vi "API - Stream - Start Data Streaming from Device.vi"(8 "error in":errorcluster, 10 "Streaming Rate (Hz)":i32, 11 "DAQiFi Device Properties In":T1) -> (0 "error out":errorcluster, 3 "DAQiFi Device Properties Out":T1)   [LabVIEW 2021]
doc: "Send a command to start the streaming of data from the DAQ device."
uses:
  TypeDefs/TypeDef - Cluster of DAQiFi Device Properties.ctl
  TypeDefs/Enum - Connection Type.ctl
  TCP - Asynchronous Write.vi
  USB - Asynchronous Write.vi
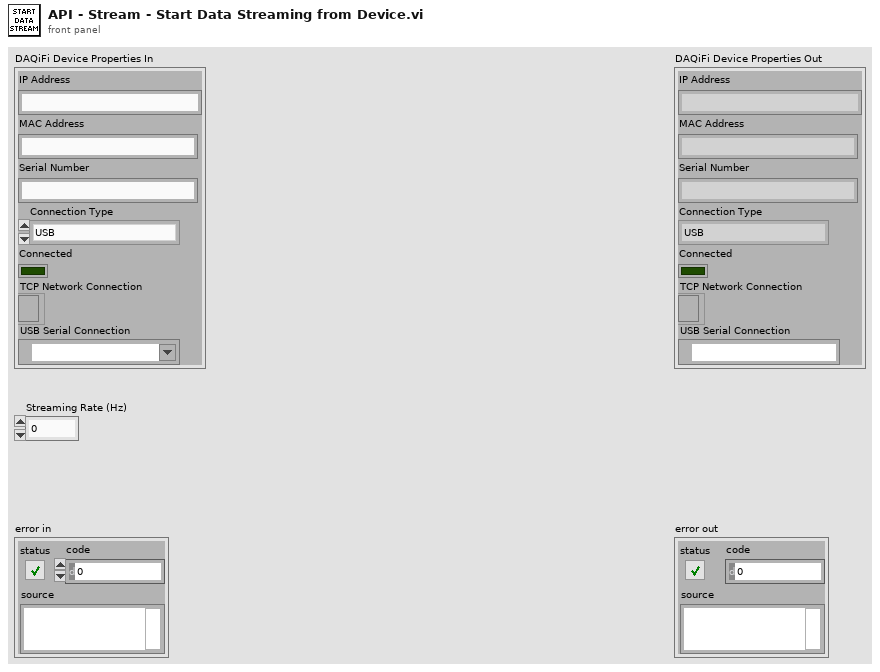
[diagram p1: front panel]
types:
  T1 = typedef "TypeDef - Cluster of DAQiFi Device Properties.ctl" = cluster{"IP Address":string, "MAC Address":string, "Serial Number":string, "Connection Type":T2, "Connected":bool, "TCP Network Connection":refnum<k5>, "USB Serial Connection":refnum<visa-resource-name>}
  T2 = typedef "Enum - Connection Type.ctl" = enum16{"USB", "TCP"}
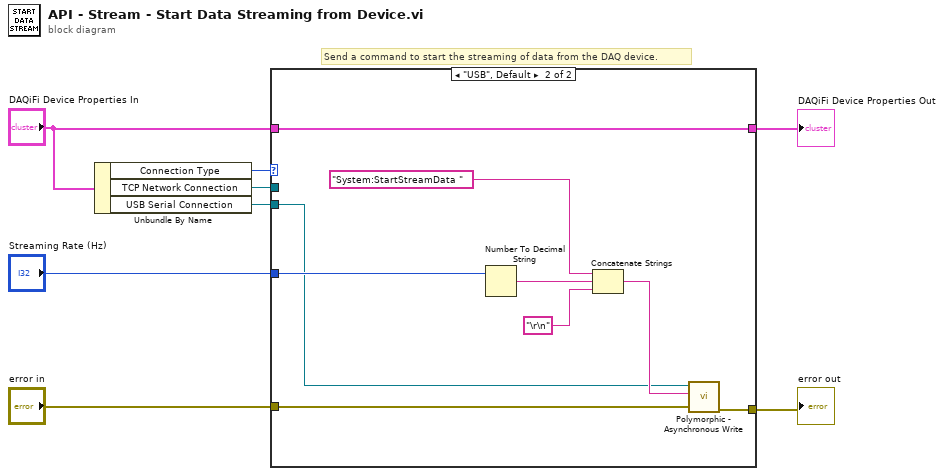
[diagram p0: block diagram]
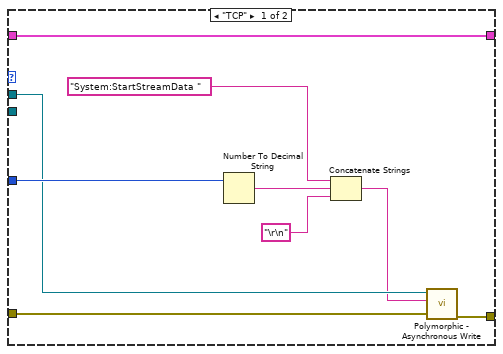
[diagram p2: hidden frame]
diagram:
  # "Send a command to start the streaming of data from the DAQ device."
  n1 = Unbundle By Name("DAQiFi Device Properties In") -> ("Connection Type"=w7:T2, "TCP Network Connection"=w4:refnum<k5>, "USB Serial Connection"=w1:refnum<visa-resource-name>)
  n2 = case shown="\"USB\", Default" w7 {
    tunnel: "Streaming Rate (Hz)" -> [w17 w26]
    tunnel: "error in" -> [w13 w22]
    tunnel: [w12 w21] -> w5
    tunnel: w4 -> [w11 _]
    tunnel: [w9 w19] -> w2
    tunnel: "DAQiFi Device Properties In" -> [w9 w19]
    tunnel: w1 -> [_ w18]
    frame "TCP" {
      n3 = Number To Decimal String(number=w17) -> (decimal integer string=w15:string)  [unwired: 1 in]
      n4 = Concatenate Strings("System:StartStreamData " ("data in"), w15, "\r\n" ("string")) -> (w10:string)
      n5 = call-poly "Polymorphic - Asynchronous Write.vi"("error in"=w13, "Message to Send"=w10, "TCP Network Connection in"=w11) -> ("error out"=w12:errorcluster)  [unwired: 7 in, 1 out]
    }
    frame "USB", Default {
      n6 = Number To Decimal String(number=w26) -> (decimal integer string=w24:string)  [unwired: 1 in]
      n7 = Concatenate Strings("System:StartStreamData " ("data in"), w24, "\r\n" ("string")) -> (w20:string)
      n8 = call-poly "Polymorphic - Asynchronous Write.vi"("error in"=w22, "Message to Send"=w20, "VISA resource name in"=w18) -> ("error out"=w21:errorcluster)  [unwired: 7 in, 1 out]
    }
  }
  "error out" <- w5
  "DAQiFi Device Properties Out" <- w2
